vi "Config Process.vi"(8 "error in (no error)":errorcluster, 11 "View Model":T1) -> (0 "error out":errorcluster)   [LabVIEW 2017]
doc: "Provides Interface of Controller to Configuration database"
uses:
  View Model/Controls/View Model.ctl
  View Model/Controls/Shared Model.ctl
  Error Handler/Controls/Error Model.ctl
  Error Handler/Controls/Error Data.ctl
  Error Handler/Controls/Error Level.ctl
  Controls/Config Model.ctl
  Controls/Config Data Record.ctl
  Controls/Config Command.ctl
  Controller/Controls/Control Model.ctl
  Controller/Controls/Elevator Location.ctl
  Controller/Controls/Elevator Status.ctl
  Controller/Controls/Control Event.ctl
  Controller/Controls/Control CMD.ctl
  Controller/Controls/Controller - Overhead.ctl
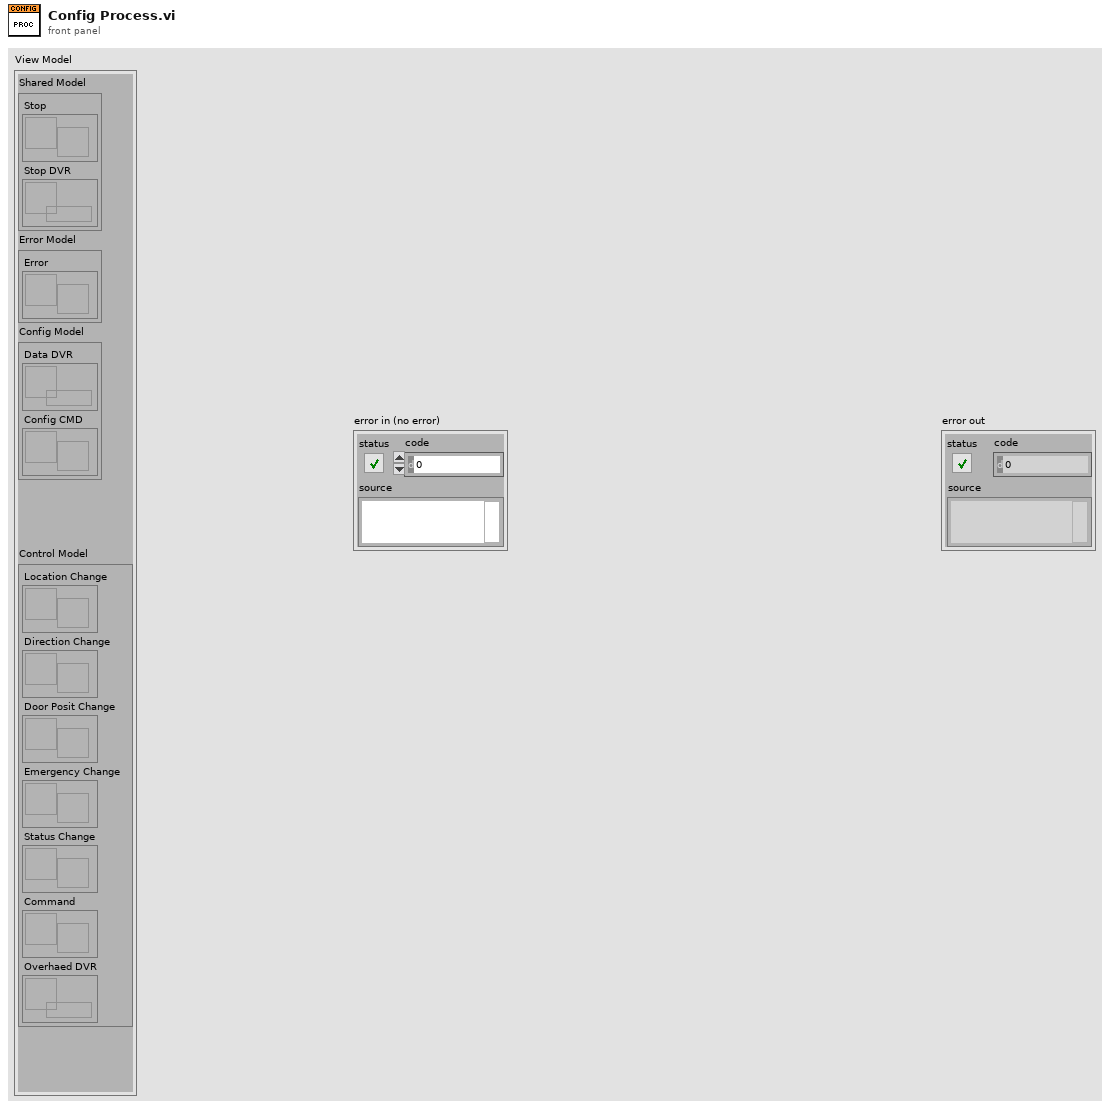
[diagram p1: front panel]
types:
  T1 = typedef "View Model.ctl" = cluster{"Shared Model":T2, "Error Model":T3, "Config Model":T4, "Control Model":T5}
  T2 = typedef "Shared Model.ctl" = cluster{"Stop":refnum<user-event>, "Stop DVR":refnum<data-value>}
  T3 = typedef "Error Model.ctl" = cluster{"Error":refnum<user-event>}
  T4 = typedef "Config Model.ctl" = cluster{"Data DVR":refnum<data-value>, "Config CMD":refnum<user-event>}
  T5 = typedef "Control Model.ctl" = cluster{"Location Change":refnum<user-event>, "Direction Change":refnum<user-event>, "Door Posit Change":refnum<user-event>, "Emergency Change":refnum<user-event>, "Status Change":refnum<user-event>, "Command":refnum<user-event>, "Overhaed DVR":refnum<data-value>}
  T6 = typedef "Config Command.ctl" = enum16{"Read", "Update"}
  T7 = typedef "Config Data Record.ctl" = cluster{"Door Open":dbl, "Door Close":dbl, "Travel Time":dbl, "Inactivity Time":dbl}
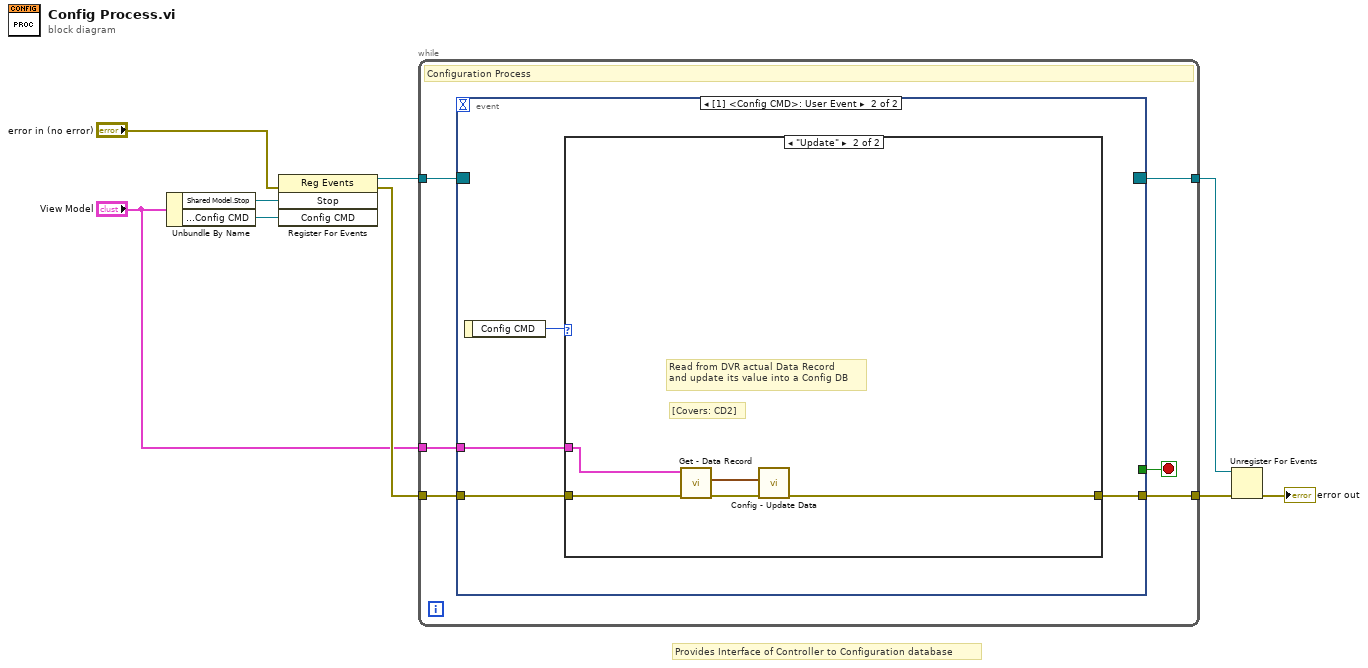
[diagram p0: block diagram]
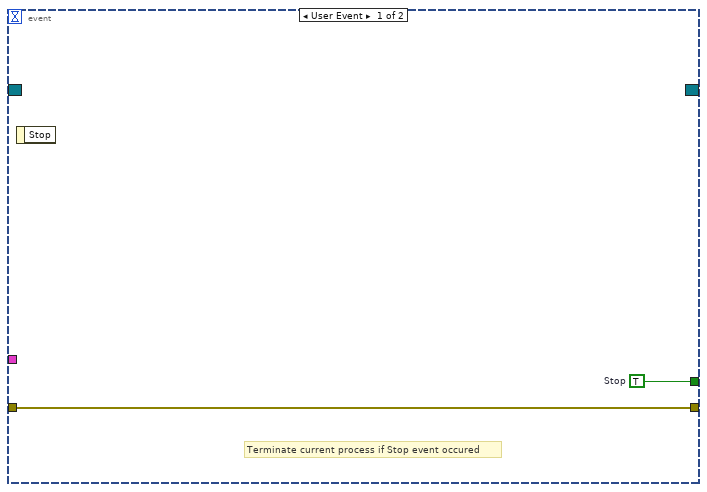
[diagram p2: hidden frame]
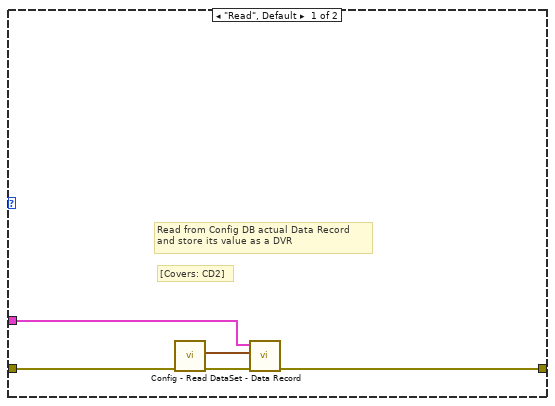
[diagram p3: hidden frame]
diagram:
  # "Provides Interface of Controller to Configuration database"
  n1 = Unbundle By Name("View Model") -> ("Shared Model.Stop"=w9:refnum<user-event>, "Config Model.Config CMD"=w2:refnum<user-event>)
  n2 = register-events(error in="error in (no error)", w9, w2) -> (reference out=w8:refnum<event-registration>, error out=w6:errorcluster)  [unwired: 1 in]
  n3 = while {
    tunnel: w8 -> [w15]
    tunnel: w6 -> [w14]
    tunnel: [w13] -> w4
    tunnel: [w11] -> w5
    tunnel: "View Model" -> [w10]
    stop <- w12 stop-if-true
    # "Configuration Process"
    n4 = event shown="[1] <Config CMD>: User Event" {
      selector: w15 -> [_ _]
      dyn-events: [_ _] -> w11
      timeout: _ -> [_ _]
      tunnel: w14 -> [w17 w19]
      tunnel: [w17 w18] -> w13
      tunnel: [w16 _] -> w12
      tunnel: w10 -> [_ w20]
      event User Event {
        w16 = TRUE  # Stop
        # "Terminate current process if Stop event occured"
        n5 = event-data() -> ()  [unwired: 1 in, 1 out]
      }
      event User Event {
        n6 = event-data() -> ("Config CMD"=w21:T6)  [unwired: 1 in]
        n7 = case shown="\"Update\"" w21 {
          tunnel: w20 -> [w26 w29]
          tunnel: w19 -> [w23 w31]
          tunnel: [w22 w27] -> w18
          frame "Read", Default {
            # "[Covers: CD2]"
            # "Read from Config DB actual Data Record\nand store its value as a DVR"
            n8 = call "Config - Read Data.vi"("error in (no error)"=w23) -> ("error out"=w25:errorcluster, "Data Record"=w24:T7)  [unwired: 9 in]
            n9 = call "Set - Data Record.vi"("error in (no error)"=w25, "Data Record"=w24, "View Model"=w26) -> ("error out"=w22:errorcluster)  [unwired: 7 in, 1 out]
          }
          frame "Update" {
            # "[Covers: CD2]"
            # "Read from DVR actual Data Record\nand update its value into a Config DB"
            n10 = call "Get - Data Record.vi"("error in (no error)"=w31, "View Model"=w29) -> ("error out"=w30:errorcluster, "Data Record"=w28:T7)  [unwired: 7 in, 1 out]
            n11 = call "Config - Update Data.vi"("error in (no error)"=w30, "Data Record"=w28) -> ("error out"=w27:errorcluster)  [unwired: 9 in]
          }
        }
      }
    }
  }
  n12 = Unregister For Events(event registration refnum=w5, error in=w4) -> (error out=→"error out":errorcluster)
